vi "Choose route.vi"(8 "robot location":dbl[](array[numeric]), 9 "target location":dbl[](array[numeric]), 10 "Map dimensions":dbl[](array[numeric]), 11 "Map":u16[][](array[ring])) -> (3 "Route":dbl[][](array[numeric]))   [LabVIEW 2015]
uses:
  <vilib>/robotics/Navigation/shared/WorldMap/OccupancyGridWorldMap/NI_Robotics_OccupancyGridWorldMap.lvclass
  <vilib>/robotics/Navigation/NI_Robotics_Navigation .lvlib
panel:
  out "Score":dbl
  out "y coordinates":i32[](array[numeric])
  out "x coordinates":i32[](array[numeric])
  out "route map":dbl[][](array[numeric])
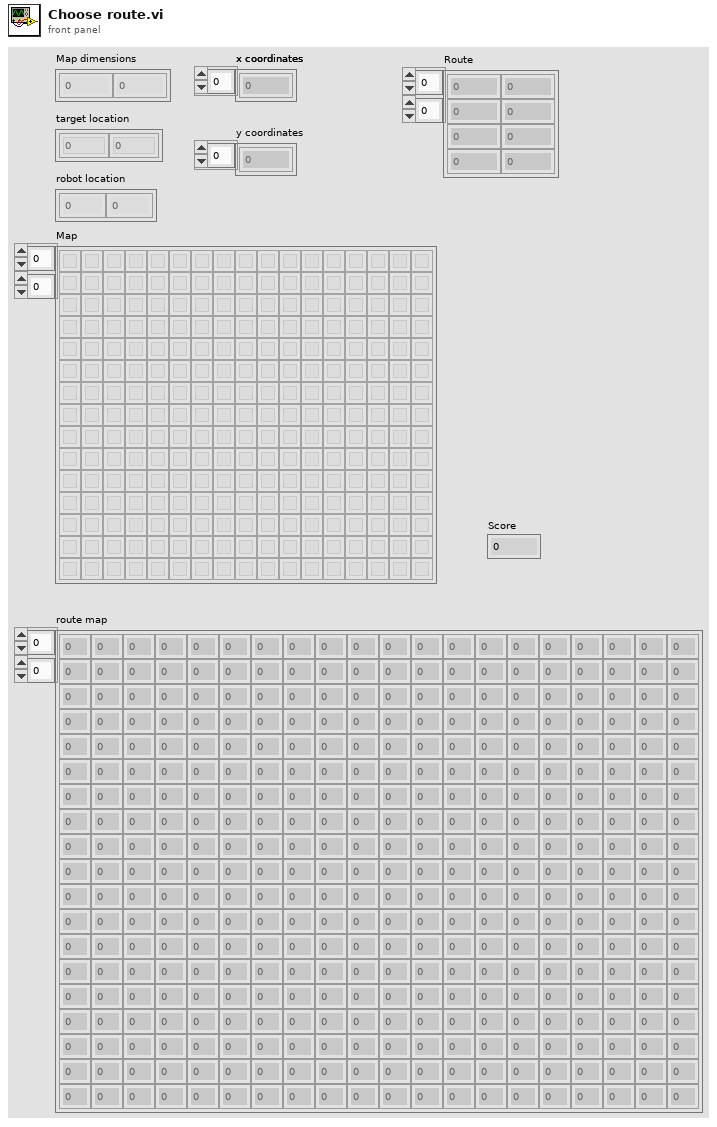
[diagram p1: front panel]
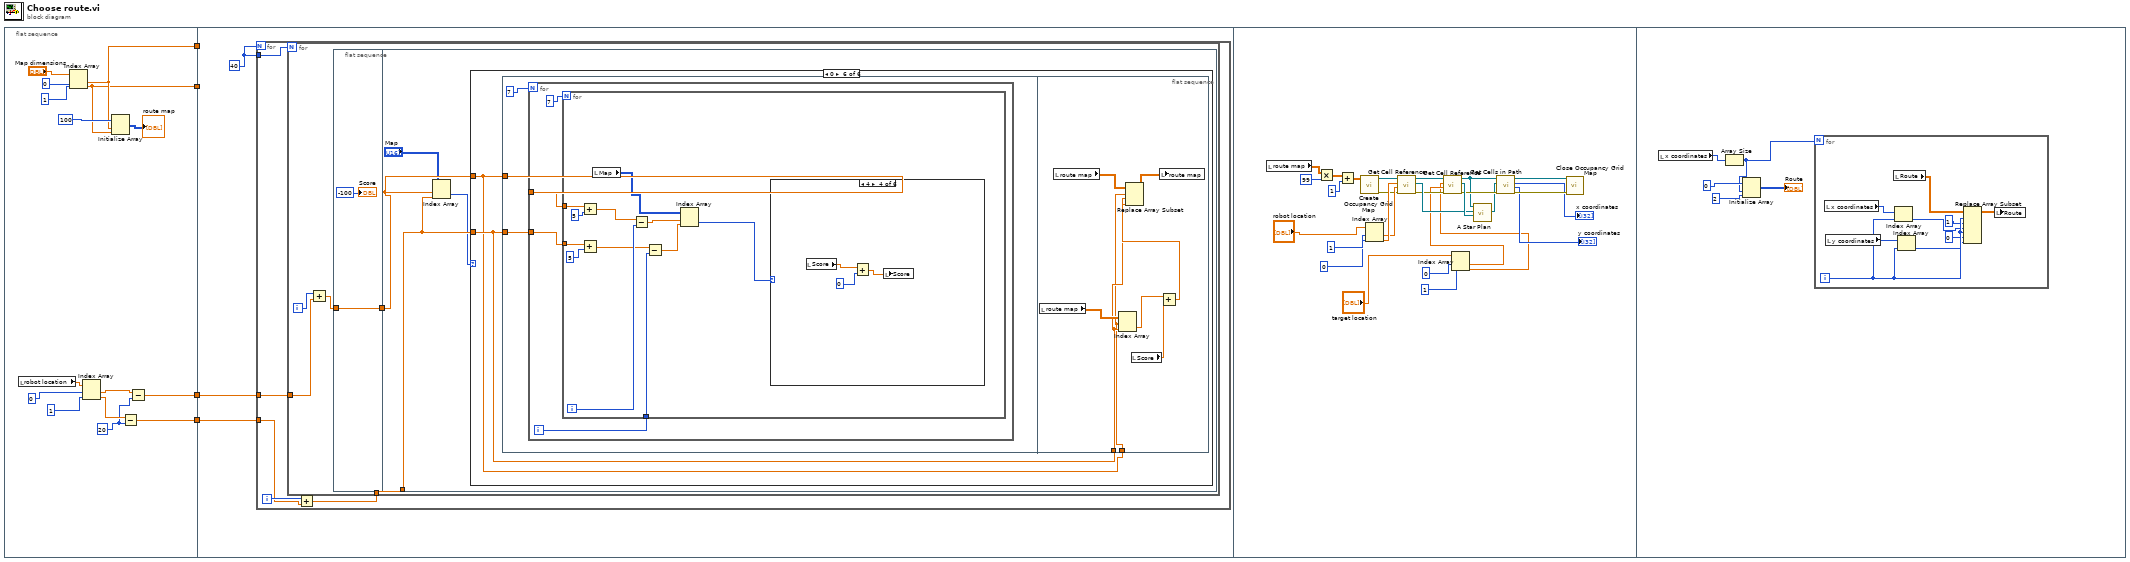
[diagram p0: block diagram]
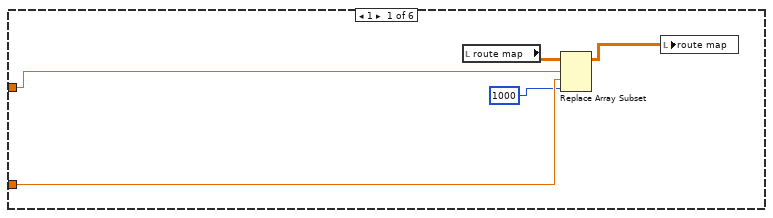
[diagram p2: hidden frame]
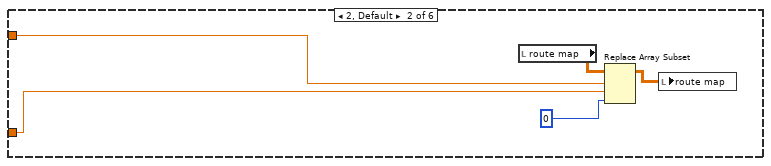
[diagram p3: hidden frame]
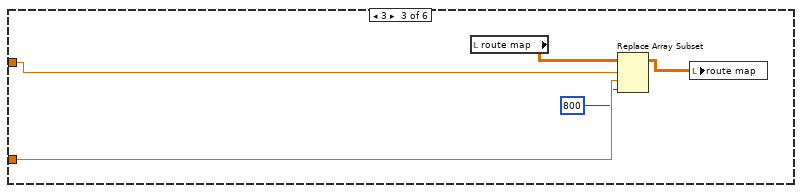
[diagram p4: hidden frame]
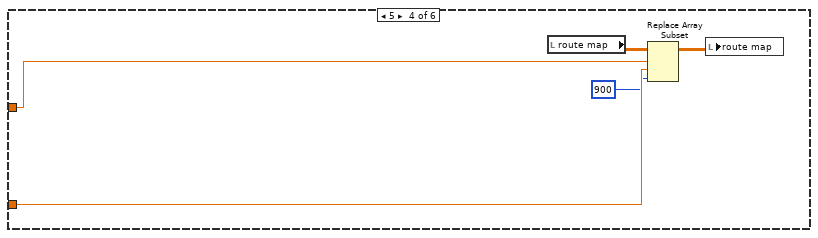
[diagram p5: hidden frame]
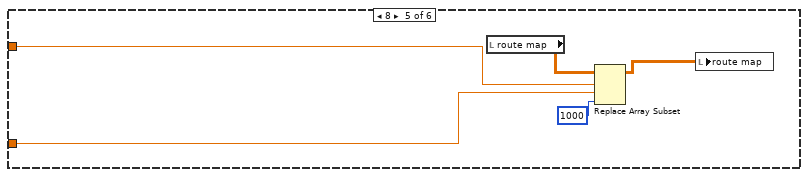
[diagram p6: hidden frame]
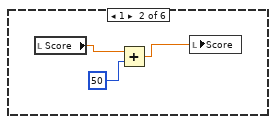
[diagram p8: hidden frame]
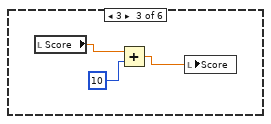
[diagram p9: hidden frame]
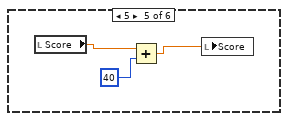
[diagram p10: hidden frame]
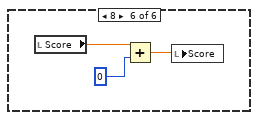
[diagram p11: hidden frame]
diagram:
  n1 = flat-sequence {
    tunnel: [w14] -> w4
    tunnel: [w13] -> w3
    tunnel: [w6] -> w2
    tunnel: [w5] -> w1
    tunnel: w4 -> [_]
    tunnel: w3 -> [_]
    tunnel: w2 -> [w22]
    tunnel: w1 -> [w21]
    frame #0 {
      w7 = 20
      n2 = local read "robot location"() -> (w12:dbl[])
      n3 = Index Array(array="Map dimensions", index #1=0, index #2=1) -> (element #1=w14:dbl, element #2=w13:dbl)
      n4 = Index Array(array=w12, index #1=0, index #2=1) -> (element #1=w9:dbl, element #2=w8:dbl)
      n5 = Initialize Array(100, w14, w13) -> (→"route map":i32[][])
      n6 = Subtract(x=w8, y=w7) -> (x-y=w6:dbl)
      n7 = Subtract(x=w9, y=w7) -> (x-y=w5:dbl)
    }
    frame #1 {
      w20 = 40
      n8 = for {
        N: w20 -> [_]
        tunnel: w22 -> [w26]
        tunnel: w21 -> [w25]
        tunnel: w20 -> [w24]
        i -> [w27]
        n9 = Add(x=w27, y=w26) -> (x+y=w23:dbl)
        n10 = for {
          N: w24 -> [_]
          tunnel: w23 -> [w32]
          tunnel: w25 -> [w28]
          i -> [w30]
          n11 = Add(x=w30, y=w28) -> (x+y=w29:dbl)
          n12 = flat-sequence {
            tunnel: w29 -> [w33]
            tunnel: [w33] -> w31
            tunnel: w32 -> [w38]
            tunnel: w31 -> [w37]
            frame #0 {
              "Score" <- -100
            }
            frame #1 {
              n13 = Index Array(array="Map", index (row)=w37, index (col)=w38) -> (element=w35:u16)
              n14 = case shown="0" w35 {
                tunnel: w38 -> [w40 w46 w50 w55 w60 w65]
                tunnel: w37 -> [w41 w45 w51 w56 w59 w64]
                frame 1 {
                  n15 = local read "route map"() -> (w43:dbl[][])
                  n16 = Replace Array Subset(array=w43, new element=1000, index (row)=w41, index (col)=w40) -> (w42:dbl[][])
                  n17 = local write "route map"(w42) -> ()
                }
                frame 2, Default {
                  n18 = local read "route map"() -> (w47:dbl[][])
                  n19 = Replace Array Subset(array=w47, new element=0, index (row)=w45, index (col)=w46) -> (w48:dbl[][])
                  n20 = local write "route map"(w48) -> ()
                }
                frame 3 {
                  n21 = local read "route map"() -> (w52:dbl[][])
                  n22 = Replace Array Subset(array=w52, new element=800, index (row)=w51, index (col)=w50) -> (w53:dbl[][])
                  n23 = local write "route map"(w53) -> ()
                }
                frame 5 {
                  n24 = local read "route map"() -> (w57:dbl[][])
                  n25 = Replace Array Subset(array=w57, new element=900, index (row)=w56, index (col)=w55) -> (w58:dbl[][])
                  n26 = local write "route map"(w58) -> ()
                }
                frame 8 {
                  n27 = local read "route map"() -> (w62:dbl[][])
                  n28 = Replace Array Subset(array=w62, new element=1000, index (row)=w59, index (col)=w60) -> (w61:dbl[][])
                  n29 = local write "route map"(w61) -> ()
                }
                frame 0 {
                  n30 = flat-sequence {
                    tunnel: w65 -> [w68]
                    tunnel: w64 -> [w67]
                    tunnel: w65 -> [w102]
                    tunnel: w64 -> [w101]
                    frame #0 {
                      n31 = for {
                        N: 7 -> [_]
                        tunnel: w68 -> [w72]
                        tunnel: w67 -> [w71]
                        i -> [w69]
                        n32 = for {
                          N: 7 -> [_]
                          tunnel: w72 -> [w81]
                          tunnel: w71 -> [w80]
                          tunnel: w69 -> [w76]
                          i -> [w78]
                          n33 = Add(x=w80, y=5) -> (x+y=w79:dbl)
                          n34 = Add(x=w81, y=5) -> (x+y=w77:dbl)
                          n35 = local read "Map"() -> (w84:u16[][])
                          n36 = Subtract(x=w79, y=w78) -> (x-y=w74:dbl)
                          n37 = Subtract(x=w77, y=w76) -> (x-y=w75:dbl)
                          n38 = Index Array(array=w84, index (row)=w74, index (col)=w75) -> (element=w73:u16)
                          n39 = case shown="4" w73 {
                            frame 0, Default {
                            }
                            frame 1 {
                              n40 = local read "Score"() -> (w86:dbl)
                              n41 = Add(x=w86, y=50) -> (x+y=w85:dbl)
                              n42 = local write "Score"(w85) -> ()
                            }
                            frame 3 {
                              n43 = local read "Score"() -> (w88:dbl)
                              n44 = Add(x=w88, y=10) -> (x+y=w89:dbl)
                              n45 = local write "Score"(w89) -> ()
                            }
                            frame 4 {
                              n46 = local read "Score"() -> (w91:dbl)
                              n47 = Add(x=w91, y=0) -> (x+y=w92:dbl)
                              n48 = local write "Score"(w92) -> ()
                            }
                            frame 5 {
                              n49 = local read "Score"() -> (w94:dbl)
                              n50 = Add(x=w94, y=40) -> (x+y=w95:dbl)
                              n51 = local write "Score"(w95) -> ()
                            }
                            frame 8 {
                              n52 = local read "Score"() -> (w98:dbl)
                              n53 = Add(x=w98, y=0) -> (x+y=w97:dbl)
                              n54 = local write "Score"(w97) -> ()
                            }
                          }
                        }
                      }
                    }
                    frame #1 {
                      n55 = local read "route map"() -> (w103:dbl[][])
                      n56 = local read "route map"() -> (w104:dbl[][])
                      n57 = Index Array(array=w103, index (row)=w101, index (col)=w102) -> (element=w106:dbl)
                      n58 = local read "Score"() -> (w100:dbl)
                      n59 = Add(x=w106, y=w100) -> (x+y=w107:dbl)
                      n60 = Replace Array Subset(array=w104, new element=w107, index (row)=w101, index (col)=w102) -> (w105:dbl[][])
                      n61 = local write "route map"(w105) -> ()
                    }
                  }
                }
              }
            }
          }
        }
      }
    }
    frame #2 {
      n62 = local read "route map"() -> (w129:dbl[][])
      n63 = Multiply(x=w129, y=99) -> (x*y=w118:dbl[][])
      n64 = Add(x=w118, y=1) -> (x+y=w120:dbl[][])
      n65 = call <vilib>:"Create Occupancy Grid Map.vi"("occupancy grid"=w120) -> ("error out"=w121:errorcluster, "map reference out"=w125:refnum<data-value>)  [unwired: 9 in]
      n66 = Index Array(array="robot location", index #1=0, index #2=1) -> (element #1=w134:dbl, element #2=w135:dbl)
      n67 = call <vilib>:"Get Cell Reference.vi"("error in (no error)"=w121, "y"=w134, "x"=w135, "map reference in"=w125) -> ("error out"=w122:errorcluster, "cell reference"=w124:refnum<data-value>, "map reference out"=w114:refnum<data-value>)  [unwired: 4 in, 1 out]
      n68 = Index Array(array="target location", index #1=0, index #2=1) -> (element #1=w109:dbl, element #2=w108:dbl)
      n69 = call <vilib>:"Get Cell Reference.vi"("error in (no error)"=w122, "y"=w109, "x"=w108, "map reference in"=w114) -> ("error out"=w123:errorcluster, "cell reference"=w126:refnum<data-value>, "map reference out"=w116:refnum<data-value>)  [unwired: 4 in, 1 out]
      n70 = call <vilib>:"A Star Plan.vi"("goal reference"=w126, "start reference"=w124, "map reference in"=w116) -> ("path references"=w115:refnum<data-value>[])  [unwired: 5 in, 3 out]
      n71 = call <vilib>:"Get Cells in Path.vi"("error in (no error)"=w123, "path references"=w115, "map reference in"=w116) -> ("error out"=w128:errorcluster, "y coordinates"=→"y coordinates":i32[], "x coordinates"=→"x coordinates":i32[], "map reference out"=w127:refnum<data-value>)  [unwired: 5 in]
      n72 = call <vilib>:"Close Occupancy Grid Map.vi"("error in (no error)"=w128, "map reference in"=w127) -> ()  [unwired: 9 in, 1 out]
    }
    frame #3 {
      n73 = local read "x coordinates"() -> (w140:i32[])
      n74 = Array Size(array=w140) -> (size(s)=w136:i32)
      n75 = Initialize Array(0, w136, 2) -> (→"Route":i32[][])
      n76 = for {
        N: w136 -> [_]
        i -> [w146]
        n77 = local read "x coordinates"() -> (w148:i32[])
        n78 = local read "y coordinates"() -> (w149:i32[])
        n79 = local read "Route"() -> (w147:dbl[][])
        n80 = Index Array(array=w148, index=w146) -> (element=w144:i32)
        n81 = Index Array(array=w149, index=w146) -> (element=w142:i32)
        n82 = Replace Array Subset(array=w147, new element #1=w144, index (row) #1=w146, index (col) #1=1, new element #2=w142, index (row) #2=w146, index (col) #2=0) -> (w141:dbl[][])
        n83 = local write "Route"(w141) -> ()
      }
    }
  }
